vi "Read configuration.vi"(8 "error in":errorcluster, 11 "RIO Target in":refnum<class "RIO Target.lvclass">) -> (0 "error out":errorcluster, 2 "configuration":refnum<class "NISE_CEF_serializable configuration.lvclass">, 3 "RIO Target out":refnum<class "RIO Target.lvclass">)   [LabVIEW 2014, in "RIO Target.lvclass"]
uses:
  RIO Target.lvclass
  <vilib>/NI/Configuration Framework/serializable configuration/NISE_CEF_serializable configuration.lvclass
  RIO Target.lvclass/RIO Target.ctl
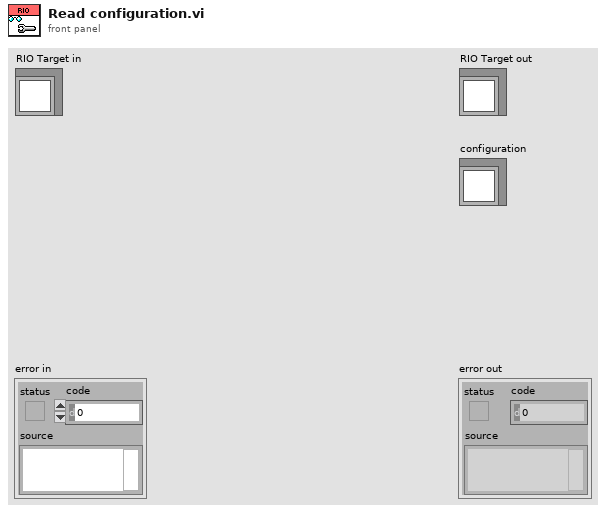
[diagram p1: front panel]
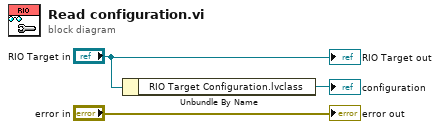
[diagram p0: block diagram]
diagram:
  n1 = Unbundle By Name("RIO Target in") -> ("RIO Target Configuration.lvclass"=→"configuration":refnum<class "RIO Target Configuration.lvclass">)
  "error out" <- "error in"
  "RIO Target out" <- "RIO Target in"
